vi "Map Display Destinations.vi"() -> (0 "Navigation Path String":string, 1 "Navigation Balloon String":string, 2 "Boundary Path String":string)   [LabVIEW 2011]
uses:
  _GlobalVariables&Libraries/ATV Program Global Variables.vi
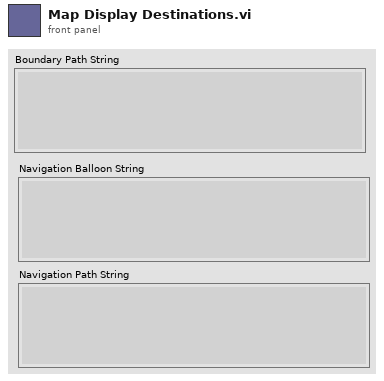
[diagram p1: front panel]
types:
  T1 = cluster{"Navigation Coordinates":cluster{"Latitude":dbl, "Longitude":dbl}[], "Coordinate Count":u32, "Drive Speed":string, "Steer Angle":dbl, "Steering":dbl, "Direction to next Coordinate":dbl, "Drive":dbl, "Navigation Path":string}
  T2 = cluster{"GPS VISA resource name":refnum<visa-resource-name>, "GPS Error":errorcluster, "Disable GPS VISA":bool, "Latitude":dbl, "Longitude":dbl, "Latitude Uncertainty":dbl, "Longitude Uncertainty":dbl, "GPS Signal":u32}
  T3 = cluster{"X":dbl, "Y":dbl, "Zoom":sgl, "Map Type":string, "Google Maps API Key":string, "Map Refresh Rate (ms)":u32, "Navigation Path Color":u32, "Navigation Path Weight":i32, "URL":string, "Boundary Coordinates":cluster{"Latitude":dbl, "Longitude":dbl}[], "GPS Balloon Character":string, "Boundary Path Color":u32, "Boundary Path Weight":i32, "GPS Balloon Size":string, "GPS Balloon Color":string, "GPS Path Color":u32, "GPS Path Weight":i32, "Disable Google Maps":bool}
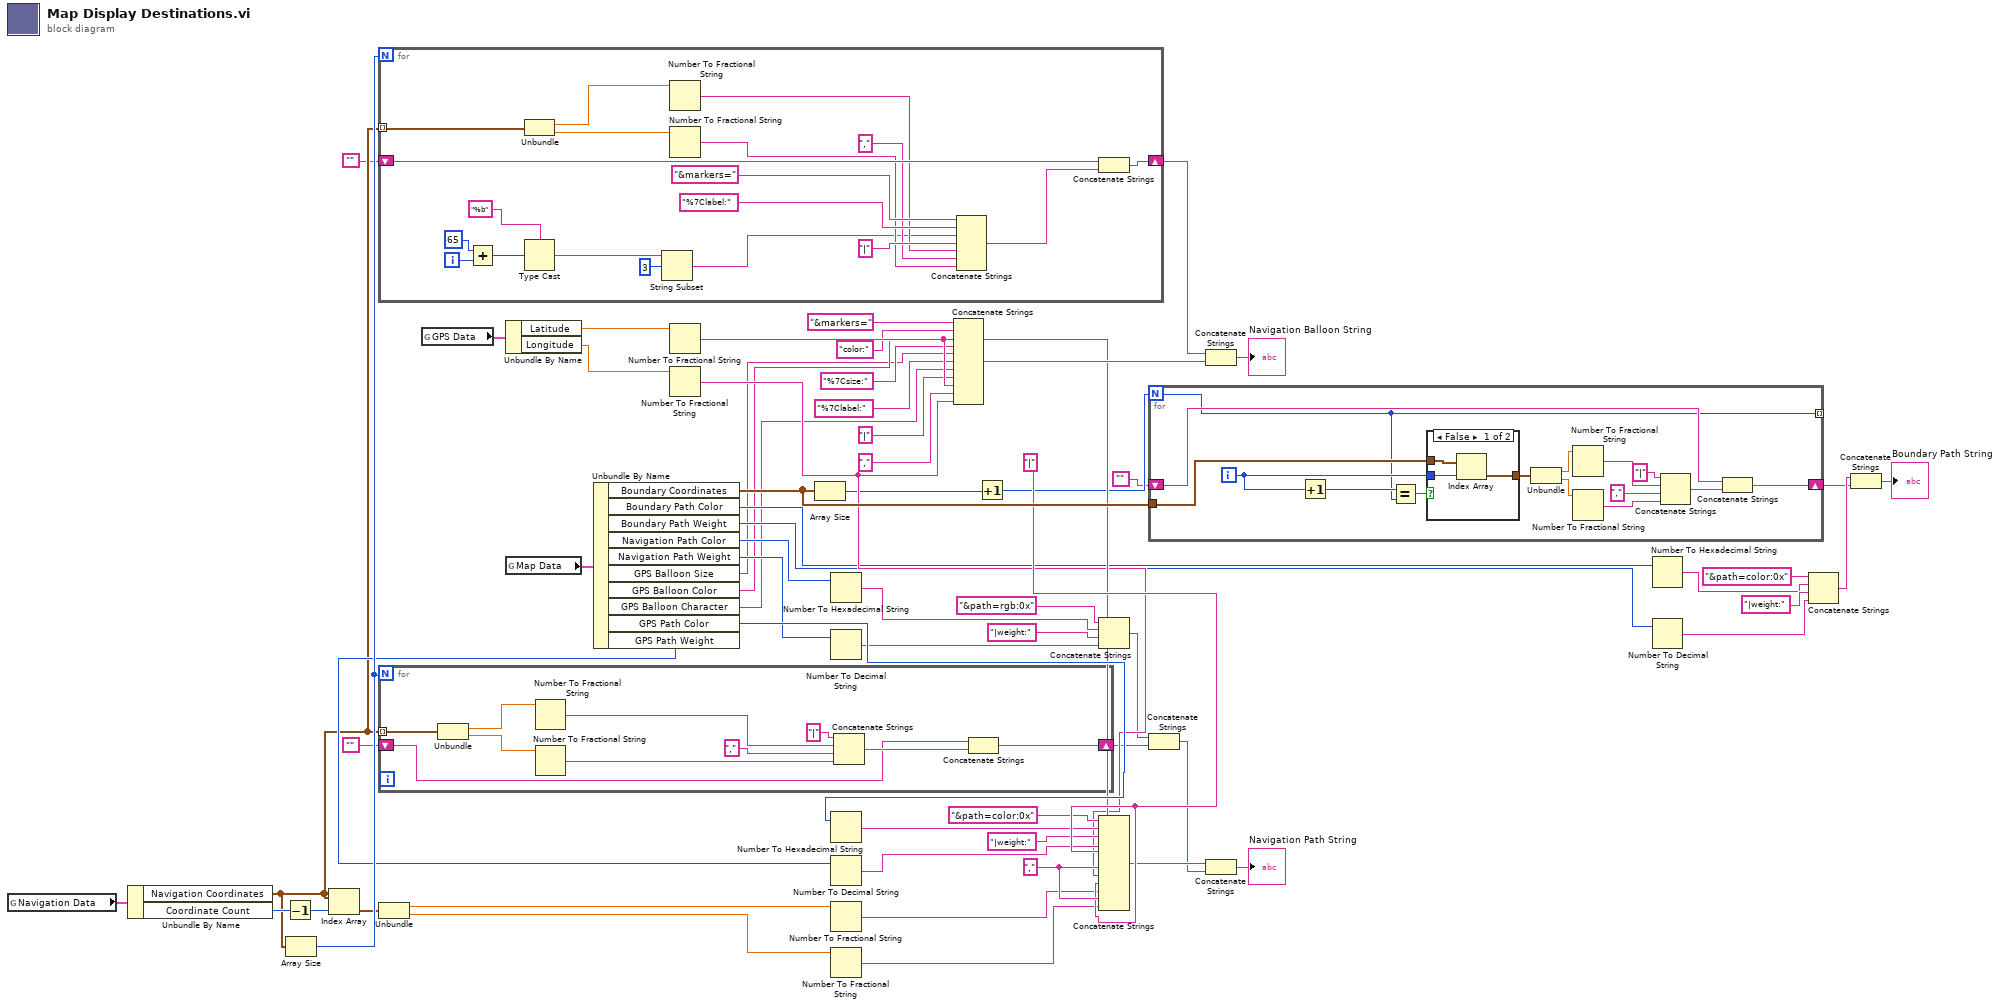
[diagram p0: block diagram]
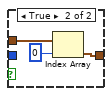
[diagram p2: hidden frame]
diagram:
  w51 = "," ("string")
  w50 = "|"
  n1 = global read "ATV Program Global Variables.vi" "Navigation Data"() -> (w61:T1)
  n2 = Unbundle By Name(w61) -> ("Navigation Coordinates"=w10:cluster{"Latitude":dbl, "Longitude":dbl}[], "Coordinate Count"=w38:u32)
  n3 = Decrement(x=w38) -> (x-1=w37:u32)
  n4 = Array Size(array=w10) -> (size(s)=w60:i32)
  n5 = Index Array(array=w10, index=w37) -> (element=w36:cluster{"Latitude":dbl, "Longitude":dbl})
  n6 = for {
    N: w60 -> [_]
    shift-right: [w80] -> w57
    shift-left: "" -> [w81]
    tunnel: w10 -> [w79] mode=indexing
    i -> [w68]
    n7 = Add(x=65, y=w68) -> (x+y=w66:i32)
    n8 = Unbundle(w79) -> ("Latitude"=w78:dbl, "Longitude"=w77:dbl)
    n9 = Type Cast(type="%b", x=w66) -> (*(type *) &x=w65:string)
    n10 = String Subset(string=w65, offset (0)=3) -> (substring=w64:string)  [unwired: 1 in]
    n11 = Number To Fractional String(number=w78) -> (F-format string=w72:string)  [unwired: 3 in]
    n12 = Number To Fractional String(number=w77) -> (F-format string=w70:string)  [unwired: 3 in]
    n13 = Concatenate Strings("&markers=", "%7Clabel:" ("string"), w64, "|" ("string"), w72, ",", w70) -> (w76:string)
    n14 = Concatenate Strings(w81, w76) -> (w80:string)
  }
  n15 = for {
    N: w60 -> [_]
    tunnel: w10 -> [w87] mode=indexing
    shift-right: [w83] -> w16
    shift-left: "" -> [w82]
    n16 = Unbundle(w87) -> ("Latitude"=w86:dbl, "Longitude"=w85:dbl)
    n17 = Number To Fractional String(number=w86) -> (F-format string=w91:string)  [unwired: 3 in]
    n18 = Number To Fractional String(number=w85) -> (F-format string=w89:string)  [unwired: 3 in]
    n19 = Concatenate Strings("|", w91, "," ("string"), w89) -> (w84:string)
    n20 = Concatenate Strings(w82, w84) -> (w83:string)
  }
  n21 = Unbundle(w36) -> ("Latitude"=w35:dbl, "Longitude"=w34:dbl)
  n22 = global read "ATV Program Global Variables.vi" "GPS Data"() -> (w58:T2)
  n23 = Unbundle By Name(w58) -> ("Latitude"=w40:dbl, "Longitude"=w39:dbl)
  n24 = global read "ATV Program Global Variables.vi" "Map Data"() -> (w62:T3)
  n25 = Unbundle By Name(w62) -> ("Boundary Coordinates"=w59:cluster{"Latitude":dbl, "Longitude":dbl}[], "Boundary Path Color"=w21:u32, "Boundary Path Weight"=w28:i32, "Navigation Path Color"=w19:u32, "Navigation Path Weight"=w18:i32, "GPS Balloon Size"=w4:string, "GPS Balloon Color"=w6:string, "GPS Balloon Character"=w2:string, "GPS Path Color"=w42:u32, "GPS Path Weight"=w41:i32)
  n26 = Number To Fractional String(number=w40) -> (F-format string=w33:string)  [unwired: 3 in]
  n27 = Number To Fractional String(number=w39) -> (F-format string=w32:string)  [unwired: 3 in]
  n28 = Array Size(array=w59) -> (size(s)=w24:i32)
  n29 = Number To Hexadecimal String(2:w19) -> (0:w12:string)  [unwired: 1 in]
  n30 = Number To Decimal String(number=w18) -> (decimal integer string=w11:string)  [unwired: 1 in]
  n31 = Number To Hexadecimal String(2:w42) -> (0:w45:string)  [unwired: 1 in]
  n32 = Number To Decimal String(number=w41) -> (decimal integer string=w47:string)  [unwired: 1 in]
  n33 = Number To Fractional String(number=w35) -> (F-format string=w49:string)  [unwired: 3 in]
  n34 = Number To Fractional String(number=w34) -> (F-format string=w48:string)  [unwired: 3 in]
  n35 = Concatenate Strings("&markers=", "color:" ("string"), w6, "%7Csize:" ("string"), w4, "%7Clabel:" ("string"), w2, "|" ("string"), w33, ",", w32) -> (w53:string)
  n36 = Increment(x=w24) -> (x+1=w25:i32)
  n37 = Concatenate Strings("&path=rgb:0x" ("string"), w12, "|weight:", w11) -> (w15:string)
  n38 = Concatenate Strings("&path=color:0x" ("string"), w45, "|weight:", w47, w50, w33, w51, w32, w50, w49, w51, w48) -> (w43:string)
  n39 = for {
    N: w25 -> [w95]
    tunnel: w59 -> [w105]
    shift-right: [w94] -> w26
    shift-left: "" -> [w98]
    tunnel: [w95] -> _ mode=indexing
    i -> [w97]
    n40 = Increment(x=w97) -> (x+1=w96:i32)
    n41 = Equal?(x=w96, y=w95) -> (x = y?=w99:bool)
    n42 = case shown="False" w99 {
      tunnel: w105 -> [w109 w112]
      tunnel: [w108 w110] -> w104
      tunnel: w97 -> [w107 _]
      frame False {
        n43 = Index Array(array=w109, index=w107) -> (element=w108:cluster{"Latitude":dbl, "Longitude":dbl})
      }
      frame True {
        n44 = Index Array(array=w112, index=0) -> (element=w110:cluster{"Latitude":dbl, "Longitude":dbl})
      }
    }
    n45 = Unbundle(w104) -> ("Latitude"=w103:dbl, "Longitude"=w102:dbl)
    n46 = Number To Fractional String(number=w103) -> (F-format string=w101:string)  [unwired: 3 in]
    n47 = Number To Fractional String(number=w102) -> (F-format string=w100:string)  [unwired: 3 in]
    n48 = Concatenate Strings("|", w101, "," ("string"), w100) -> (w93:string)
    n49 = Concatenate Strings(w98, w93) -> (w94:string)
  }
  n50 = Concatenate Strings(w15, w16) -> (w17:string)
  n51 = Concatenate Strings(w57, w53) -> (→"Navigation Balloon String":string)
  n52 = Concatenate Strings(w43, w17) -> (→"Navigation Path String":string)
  n53 = Number To Hexadecimal String(2:w21) -> (0:w20:string)  [unwired: 1 in]
  n54 = Number To Decimal String(number=w28) -> (decimal integer string=w30:string)  [unwired: 1 in]
  n55 = Concatenate Strings("&path=color:0x" ("string"), w20, "|weight:", w30) -> (w27:string)
  n56 = Concatenate Strings(w27, w26) -> (→"Boundary Path String":string)
